vi "IO-4 Bricklet Test.vi"() -> ()   [LabVIEW 2011]
uses:
  Classes/IP Connection/IP Connection.lvclass
  Classes/IO-4 Bricklet/IO-4 Bricklet.lvclass
panel:
  out "appended array":bool[](array[boolean])
  out "x-y":u32
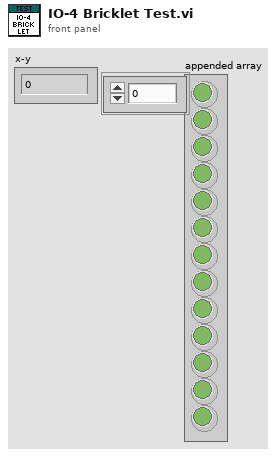
[diagram p1: front panel]
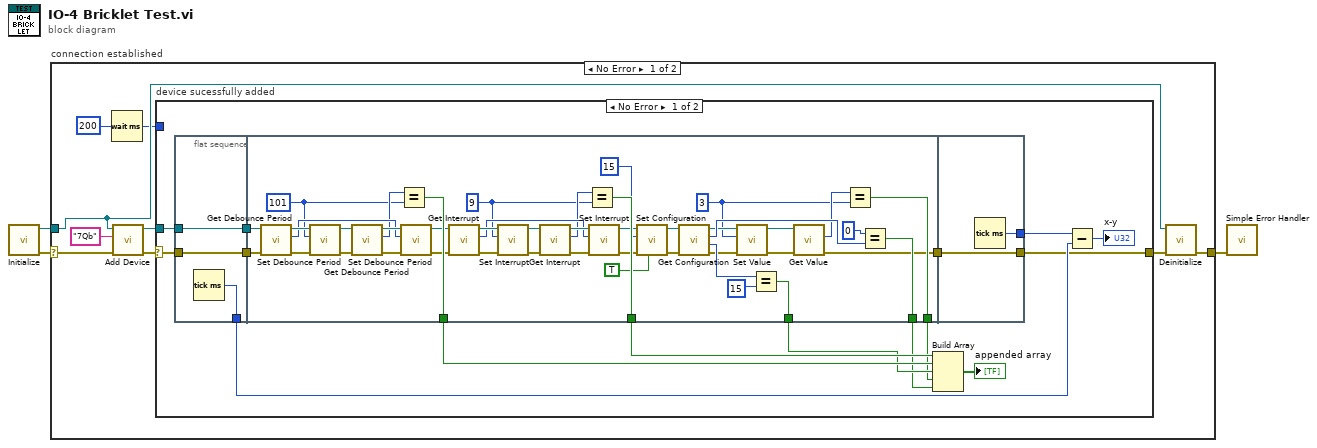
[diagram p0: block diagram]
diagram:
  n1 = call "Initialize.vi"() -> ("error out"=w1:errorcluster, "IP Connection out"=w3:refnum<class "IP Connection.lvclass">)  [unwired: 10 in]
  n2 = case "connection established" shown="No Error" w1 {
    selector: w1 -> [w8 w78]
    tunnel: w3 -> [w12 _]
    tunnel: [w4 w78] -> w2
    frame No Error {
      n3 = Wait (ms)(milliseconds to wait=u32 200) -> (millisecond timer value=w5:u32)
      n4 = call "Add Device.vi"("Error In"=w8, "Device UID"="7Qb", "IP Connection"=w12) -> ("Error Out"=w7:errorcluster, "IO-4 Bricklet"=w9:refnum<class "IO-4 Bricklet.lvclass">)  [unwired: 7 in]
      n5 = case "device sucessfully added" shown="No Error" w7 {
        selector: w7 -> [w27 w77]
        tunnel: [w13 w77] -> w10
        tunnel: w9 -> [w26 _]
        tunnel: w5 -> [_ _]
        frame No Error {
          n6 = flat-sequence {
            tunnel: w26 -> [w29]
            tunnel: w27 -> [w30]
            tunnel: [w30] -> w24
            tunnel: [w29] -> w23
            tunnel: [w28] -> w21
            tunnel: [w31] -> w25
            tunnel: w24 -> [w74]
            tunnel: w23 -> [w73]
            tunnel: [w51] -> w19
            tunnel: [w63] -> w18
            tunnel: [w40] -> w17
            tunnel: [w32] -> w16
            tunnel: [w39] -> w15
            tunnel: [w76] -> w13
            tunnel: w25 -> [w76]
            tunnel: [w75] -> w22
            frame #0 {
              n7 = Tick Count (ms)() -> (millisecond timer value=w28:u32)
            }
            frame #1 {
              w33 = u8 3 ("Value Mask")
              w52 = u8 9 ("Interrupt Mask")
              w64 = u32 101 ("debounce (100)")
              n8 = call "Get Debounce Period.vi"("error in (no error)"=w74, "IO-4 Bricklet in"=w73) -> ("error out"=w72:errorcluster, "debounce"=w66:u32, "IO-4 Bricklet out"=w71:refnum<class "IO-4 Bricklet.lvclass">)  [unwired: 7 in]
              n9 = call "Set Debounce Period.vi"("error in (no error)"=w72, "debounce (100)"=w64, "IO-4 Bricklet in"=w71) -> ("error out"=w69:errorcluster, "IO-4 Bricklet out"=w68:refnum<class "IO-4 Bricklet.lvclass">)  [unwired: 7 in]
              n10 = call "Get Debounce Period.vi"("error in (no error)"=w69, "IO-4 Bricklet in"=w68) -> ("error out"=w67:errorcluster, "debounce"=w65:u32, "IO-4 Bricklet out"=w70:refnum<class "IO-4 Bricklet.lvclass">)  [unwired: 7 in]
              n11 = Equal?(x=w65, y=w64) -> (x = y?=w63:bool)
              n12 = call "Set Debounce Period.vi"("error in (no error)"=w67, "debounce (100)"=w66, "IO-4 Bricklet in"=w70) -> ("error out"=w62:errorcluster, "IO-4 Bricklet out"=w61:refnum<class "IO-4 Bricklet.lvclass">)  [unwired: 7 in]
              n13 = call "Get Interrupt.vi"("error in (no error)"=w62, "IO-4 Bricklet in"=w61) -> ("error out"=w60:errorcluster, "Interrupt Mask"=w54:u8, "IO-4 Bricklet out"=w59:refnum<class "IO-4 Bricklet.lvclass">)  [unwired: 7 in]
              n14 = call "Set Interrupt.vi"("error in (no error)"=w60, "Interrupt Mask"=w52, "IO-4 Bricklet in"=w59) -> ("error out"=w57:errorcluster, "IO-4 Bricklet out"=w56:refnum<class "IO-4 Bricklet.lvclass">)  [unwired: 7 in]
              n15 = call "Get Interrupt.vi"("error in (no error)"=w57, "IO-4 Bricklet in"=w56) -> ("error out"=w58:errorcluster, "Interrupt Mask"=w53:u8, "IO-4 Bricklet out"=w55:refnum<class "IO-4 Bricklet.lvclass">)  [unwired: 7 in]
              n16 = Equal?(x=w53, y=w52) -> (x = y?=w51:bool)
              n17 = call "Set Interrupt.vi"("error in (no error)"=w58, "Interrupt Mask"=w54, "IO-4 Bricklet in"=w55) -> ("error out"=w50:errorcluster, "IO-4 Bricklet out"=w49:refnum<class "IO-4 Bricklet.lvclass">)  [unwired: 7 in]
              n18 = call "Set Configuration.vi"("Value"=TRUE, "error in (no error)"=w50, "Pin Mark"=u8 15, "IO-4 Bricklet in"=w49) -> ("error out"=w46:errorcluster, "IO-4 Bricklet out"=w45:refnum<class "IO-4 Bricklet.lvclass">)  [unwired: 6 in]
              n19 = call "Get Configuration.vi"("error in (no error)"=w46, "IO-4 Bricklet in"=w45) -> ("error out"=w38:errorcluster, "Value Mask"=w42:u8, "Direction Mask"=w44:u8, "IO-4 Bricklet out"=w37:refnum<class "IO-4 Bricklet.lvclass">)  [unwired: 6 in]
              n20 = call "Set Value.vi"("error in (no error)"=w38, "Value Mask"=w33, "IO-4 Bricklet in"=w37) -> ("error out"=w36:errorcluster, "IO-4 Bricklet out"=w35:refnum<class "IO-4 Bricklet.lvclass">)  [unwired: 7 in]
              n21 = Equal?(x=w42, y=u8 15) -> (x = y?=w40:bool)
              n22 = call "Get Value.vi"("error in (no error)"=w36, "IO-4 Bricklet in"=w35) -> ("error out"=w31:errorcluster, "Value Mask"=w34:u8)  [unwired: 7 in, 1 out]
              n23 = Equal?(x=w34, y=w33) -> (x = y?=w32:bool)
              n24 = Equal?(x=u8 0, y=w44) -> (x = y?=w39:bool)
            }
            frame #2 {
              n25 = Tick Count (ms)() -> (millisecond timer value=w75:u32)
            }
          }
          n26 = Build Array(w19, w18, w17, w16, w15) -> (→"appended array":bool[])
          n27 = Subtract(x=w22, y=w21) -> (x-y=→"x-y":u32)
        }
        frame Error {
        }
      }
      n28 = call "Deinitialize.vi"("error in (no error)"=w10, "IP Connection in"=w12) -> ("error out"=w4:errorcluster)  [unwired: 9 in]
    }
    frame Error {
    }
  }
  n29 = call <vilib>:"Simple Error Handler.vi"("error in (no error)"=w2) -> ()  [unwired: 4 in, 5 out]
